vi "Create.vi"(8 "error in":errorcluster, 10 "gRPC ID in":T1) -> (0 "error out":errorcluster, 2 "gRPC ID out":T1, 3 "measurement service out":refnum<class "IMeasurement Service.lvclass">)   [LabVIEW 2020, in "Measurement Plugin Measurement Server.lvlib" / "Measurement Service V2.lvclass"]
uses:
  Measurement Service V2.lvclass
  IMeasurement Service/IMeasurement Service.lvclass
  <vilib>/gRPC/LabVIEW gRPC Library/Shared/grpcId.ctl
  gRPC/Generated APIs/ni/measurementlink/measurement/v2/RPC Service/MeasurementService/MeasurementServiceBaseV2.lvclass
  C:/dev/measurementlink-labview/Source/Runtime/Measurements/Measurement Plugin Measurement Server/IMeasurement Service/IMeasurement Service.lvclass
  Measurement Service V2.lvclass/Measurement Service V2.ctl
  <vilib>/gRPC/LabVIEW gRPC Library/grpc-lvsupport-release.lvlib
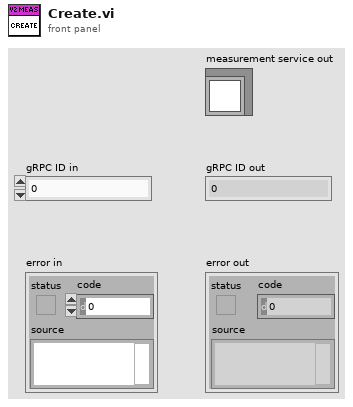
[diagram p1: front panel]
types:
  T1 = typedef "grpc-lvsupport-release.lvlib/grpcId.ctl" = u64
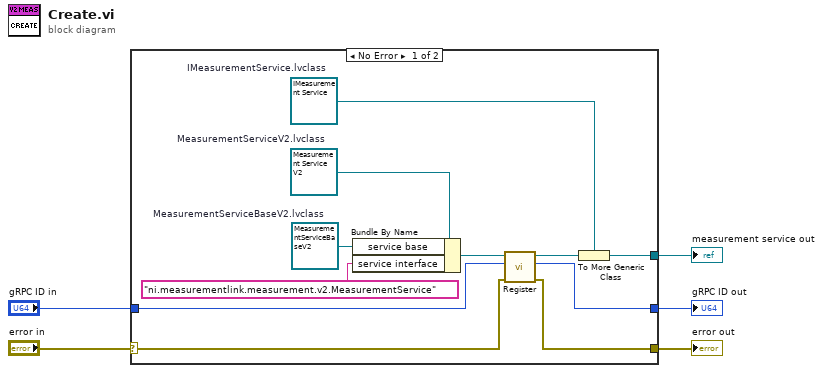
[diagram p0: block diagram]
diagram:
  n1 = case shown="No Error" "error in" {
    selector: "error in" -> [w8 w18]
    tunnel: [w7 w18] -> w4
    tunnel: [w14 _] -> w3
    tunnel: "gRPC ID in" -> [w9 w17]
    tunnel: [w6 w17] -> w1
    frame No Error {
      w12 = refnum<class "Measurement Service V2.lvclass"> refnum  # MeasurementServiceV2.lvclass
      w13 = refnum<class "IMeasurement Service.lvclass"> refnum  # IMeasurementService.lvclass
      w16 = refnum<class "MeasurementServiceBaseV2.lvclass"> refnum  # MeasurementServiceBaseV2.lvclass
      n2 = Bundle By Name(cluster=w12, "service base"=w16, "service interface"="ni.measurementlink.measurement.v2.MeasurementService") -> (w11:refnum<class "Measurement Service V2.lvclass">)
      n3 = call "Register.vi"("error in"=w8, "gRPC ID in"=w9, "measurement service v2 in"=w11) -> ("error out"=w7:errorcluster, "gRPC ID out"=w6:T1, "measurement service v2 out"=w10:refnum<class "Measurement Service V2.lvclass">)  [unwired: 6 in]
      n4 = To More Generic Class(target class=w13, reference=w10) -> (generic class reference=w14:refnum<class "IMeasurement Service.lvclass">)
    }
    frame Error {
    }
  }
  "error out" <- w4
  "measurement service out" <- w3
  "gRPC ID out" <- w1
